vi "ILAB_ShowStatus.vi"(1 "Time Remaining":string, 2 "Status":string) -> ()   [LabVIEW 2009]
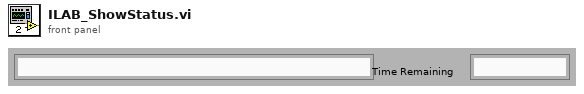
[diagram p1: front panel]
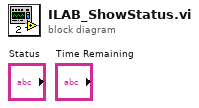
[diagram p0: block diagram]
diagram:
